vi "unpack2bytes.vi"(1 "ID":u16[](array[numeric])=[16, 32] format="%x") -> (0 "number":u16)   [LabVIEW 2020]
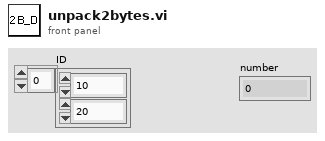
[diagram p1: front panel]
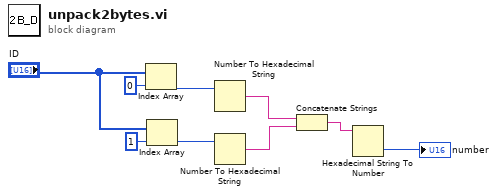
[diagram p0: block diagram]
diagram:
  n1 = Index Array(array="ID", index=0) -> (element=w7:u16)
  n2 = Index Array(array="ID", index=1) -> (element=w6:u16)
  n3 = Number To Hexadecimal String(2:w7) -> (0:w5:string)  [unwired: 1 in]
  n4 = Number To Hexadecimal String(2:w6) -> (0:w4:string)  [unwired: 1 in]
  n5 = Concatenate Strings(w5, w4) -> (w3:string)
  n6 = Hexadecimal String To Number(string=w3) -> (number=→"number":u32)  [unwired: 2 in, 1 out]
